vi "uTTA_SetPGAGain.vi"(5 "Mode":T1, 8 "error in":errorcluster, 10 "PGA Gain":u16 max=3, 11 "VISA Refnum in":refnum<visa-resource-name>) -> (0 "error out":errorcluster, 3 "VISA Refnum out":refnum<visa-resource-name>, 4 "Set PGA Gain":u32, 7 "Received":string)   [LabVIEW 2021]
uses:
  CTL_uTTA_PGA_Gain.ctl
panel:
  out "Heating PGA Gain":u32
  out "Cooling PGA Gain":u32
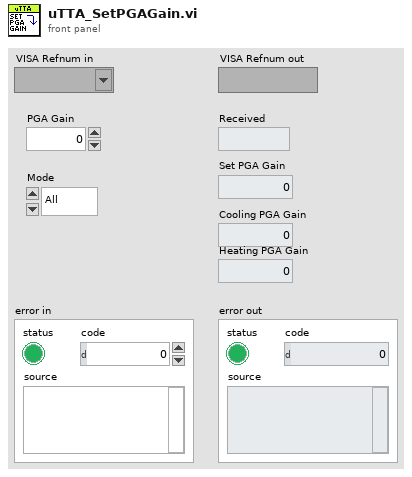
[diagram p1: front panel]
types:
  T1 = typedef "CTL_uTTA_PGA_Gain.ctl" = enum16{"All", "Cooling", "Heating"}
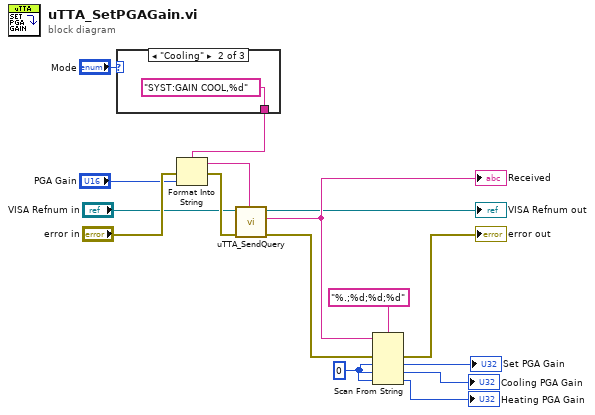
[diagram p0: block diagram]
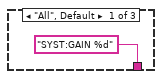
[diagram p2: hidden frame]
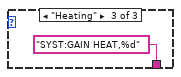
[diagram p3: hidden frame]
diagram:
  w3 = u32 0 ("default value 1")
  n1 = case shown="\"Cooling\"" "Mode" {
    tunnel: ["SYST:GAIN %d" ("format string") "SYST:GAIN COOL,%d" ("format string") "SYST:GAIN HEAT,%d" ("format string")] -> w4
    frame "All", Default {
    }
    frame "Cooling" {
    }
    frame "Heating" {
    }
  }
  n2 = Format Into String(format string=w4, error in="error in", "PGA Gain") -> (resulting string=w10:string, error out=w12:errorcluster)  [unwired: 1 in]
  n3 = call "uTTA_SendQuery.vi"("Send String"=w10, "error in (no error)"=w12, "VISA Refnum in"="VISA Refnum in") -> ("error out"=w15:errorcluster, "Received"=w13:string, "VISA Refnum out"=→"VISA Refnum out":refnum<visa-resource-name>)  [unwired: 6 in]
  "Received" <- w13
  n4 = Scan From String(format string="%.;%d;%d;%d", input string=w13, error in=w15, default 1=w3, default 2=w3, default 3=w3) -> (error out=→"error out":errorcluster, output 1=→"Set PGA Gain":u32, output 2=→"Cooling PGA Gain":u32, output 3=→"Heating PGA Gain":u32)  [unwired: 1 in, 2 out]
